vi "Get Controller Variables Ranges.vi"(8 "error in (no error)":errorcluster, 10 "Path":string, 11 "NIVS.SysDef Ref":refnum<k24>) -> (0 "error out":errorcluster, 2 "Diagnostic Protocol":T1)   [LabVIEW 2015, in "Diagnostics Addon Shared.lvlib"]
uses:
  NationalInstruments.VeriStand.SystemStorage
  Types/Diagnostic Protocols.ctl
  NationalInstruments.VeriStand
  GUID Lookup.vi
  Diagnostics Addon Shared.lvlib
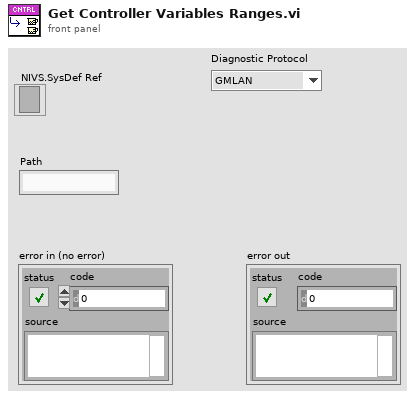
[diagram p1: front panel]
types:
  T1 = typedef "Diagnostics Addon Shared.lvlib/Diagnostic Protocols.ctl" = enum16{"GMLAN", "KWP-2000", "UDS"}
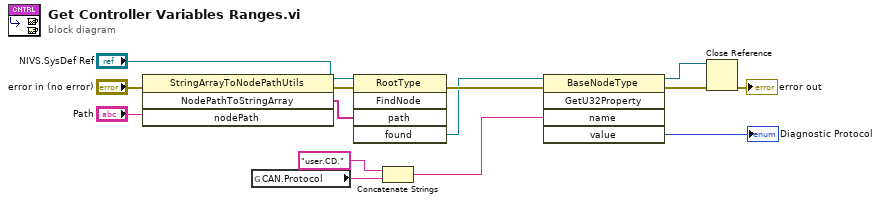
[diagram p0: block diagram]
diagram:
  n1 = invoke class="StringArrayToNodePathUtils" method="NodePathToStringArray"(error in="error in (no error)", "nodePath"="Path") -> (error out=w9:errorcluster, "NodePathToStringArray"=w11:string[])  [unwired: 2 in, 2 out]
  n2 = global read "GUID Lookup.vi" "CAN.Protocol"() -> (w14:string)
  n3 = invoke class="RootType" method="FindNode"(reference="NIVS.SysDef Ref", error in=w9, "path"=w11) -> (error out=w13:errorcluster, "found"=w6:refnum<k24>)  [unwired: 2 in, 3 out]
  n4 = Concatenate Strings("user.CD." ("string"), w14) -> (w4:string)
  n5 = invoke class="BaseNodeType" method="GetU32Property"(reference=w6, error in=w13, "name"=w4) -> (reference out=w2:refnum<k24>, error out=w3:errorcluster, "value"=→"Diagnostic Protocol":u32)  [unwired: 2 in, 2 out]
  n6 = Close Reference(reference=w2, error in (no error)=w3) -> (error out=→"error out":errorcluster)
